vi "Check Alignment.vi"(8 "Current State":T1=enum."Turn Tote Right", 10 "Right Pot":dbl, 11 "Left Pot":dbl) -> (3 "State Output":T1=enum."Turn Tote Right")   [LabVIEW 2014]
uses:
  Common Code/Inner Roller States.ctl
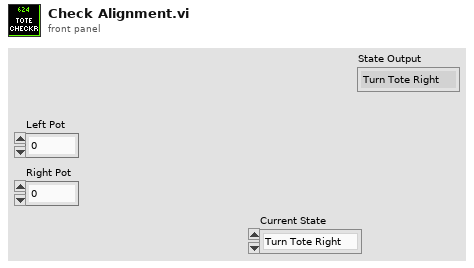
[diagram p1: front panel]
types:
  T1 = typedef "Inner Roller States.ctl" = enum16{"Turn Tote Portrait", "Acquire Tote", "Absorb Tote", "Turn Tote Right", "Turn Tote Left"}
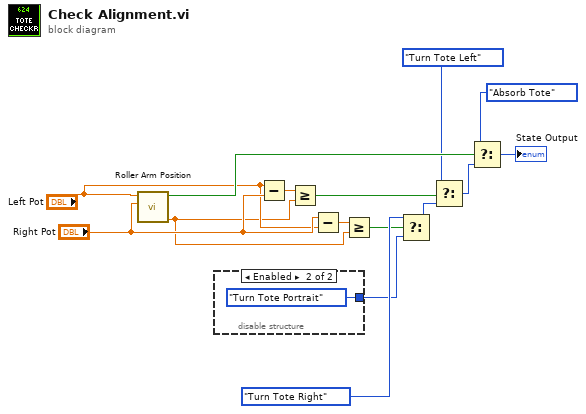
[diagram p0: block diagram]
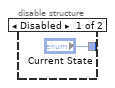
[diagram p2: hidden frame]
diagram:
  n1 = call "Roller Arm Position.vi"("Right Pot"="Right Pot", "Left Pot"="Left Pot") -> ("Pot Diff"=w1:dbl, "Portrait?"=w15:bool)  [unwired: 6 in, 2 out]
  n2 = disable-structure shown="Enabled" {
    disable-tunnel: ["Current State" Inner_Roller_States."Turn Tote Portrait" ("Current State")] -> w8
    frame Disabled {
    }
    frame Enabled {
    }
  }
  n3 = Subtract(x="Left Pot", y="Right Pot") -> (x-y=w7:dbl)
  n4 = Greater Or Equal?(x=w7, y=w1) -> (x >= y?=w6:bool)
  n5 = Subtract(x="Right Pot", y="Left Pot") -> (x-y=w5:dbl)
  n6 = Greater Or Equal?(x=w5, y=w1) -> (x >= y?=w4:bool)
  n7 = Select(t=Inner_Roller_States."Turn Tote Right" ("Enum"), s=w4, f=w8) -> (s? t:f=w13:T1)
  n8 = Select(t=Inner_Roller_States."Turn Tote Left" ("Enum"), s=w6, f=w13) -> (s? t:f=w11:T1)
  n9 = Select(t=Inner_Roller_States."Absorb Tote" ("Enum"), s=w15, f=w11) -> (s? t:f=→"State Output":T1)
